vi "Black_image_detection.vi"(0 "Match score":i32[](array[numeric])) -> (1 "No Error":bool)   [LabVIEW 2024]
doc: "Compares the match score from the computer vision to determine if the image were taken with or without errors."
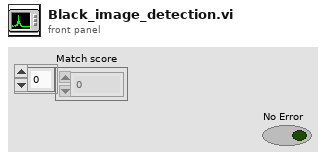
[diagram p1: front panel]
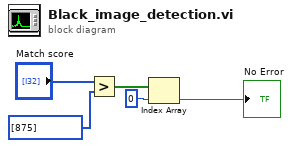
[diagram p0: block diagram]
diagram:
  n1 = Greater?(x="Match score", y=i32[] [875]) -> (0:w3:bool[])
  n2 = Index Array(array=w3, index=0) -> (element=→"No Error":bool)
